vi "vibratome3 waveform gen.vi"(8 "error in":errorcluster, 9 "frequency(HZ)":dbl format="%#_13g", 10 "slice time":dbl format="%#_13g", 11 "ramp time(s)":dbl format="%#_13g") -> (0 "error out":errorcluster, 2 "vib wave":dbl[](graph))   [LabVIEW 2018]
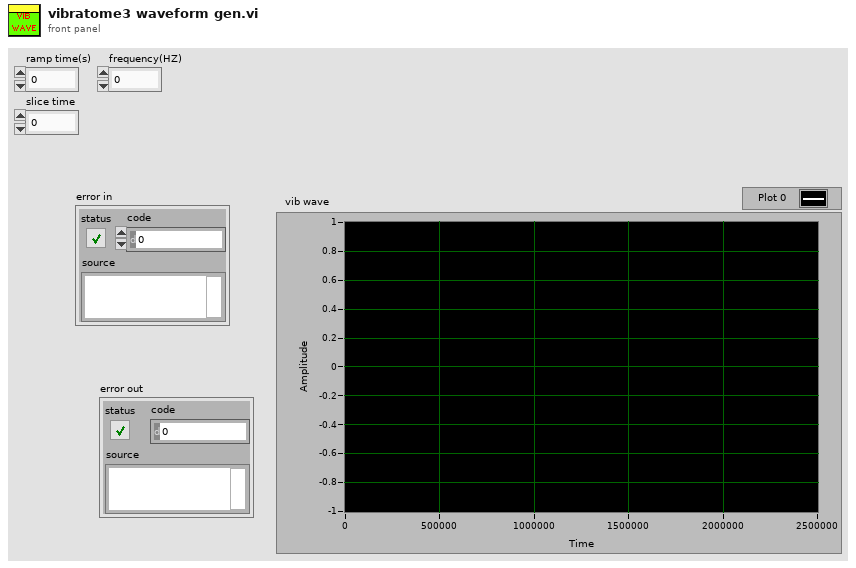
[diagram p1: front panel]
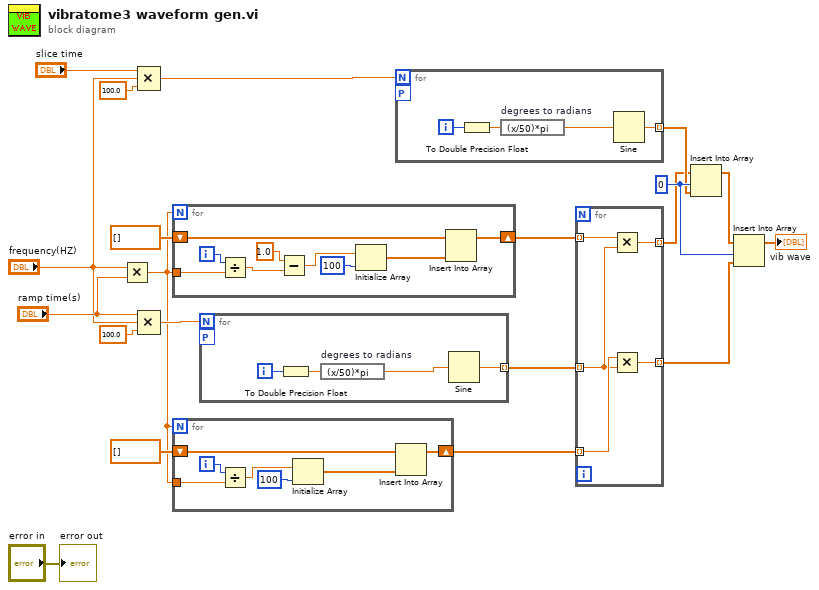
[diagram p0: block diagram]
diagram:
  w6 = 0 ("index")
  n1 = Multiply(x="frequency(HZ)", y="ramp time(s)") -> (x*y=w8:dbl)
  n2 = Compound Arithmetic op=MULTIPLY("slice time", "frequency(HZ)", 100.0) -> (w14:dbl)
  n3 = Compound Arithmetic op=MULTIPLY("ramp time(s)", "frequency(HZ)", 100.0) -> (w19:dbl)
  n4 = for {
    N: w8 -> [_]
    tunnel: w8 -> [w28]
    shift-right: [w24] -> w10
    shift-left: dbl[] [] -> [w25]
    i -> [w29]
    n5 = Divide(x=w29, y=w28) -> (x/y=w21:dbl)
    n6 = Subtract(x=1.0, y=w21) -> (x-y=w23:dbl)
    n7 = Initialize Array(w23, 100 ("dimension size")) -> (w26:dbl[])
    n8 = Insert Into Array(array=w25, new element=w26) -> (w24:dbl[])  [unwired: 1 in]
  }
  n9 = for {
    N: w8 -> [_]
    tunnel: w8 -> [w35]
    shift-right: [w30] -> w11
    shift-left: dbl[] [] -> [w31]
    i -> [w36]
    n10 = Divide(x=w36, y=w35) -> (x/y=w34:dbl)
    n11 = Initialize Array(w34, 100 ("dimension size")) -> (w32:dbl[])
    n12 = Insert Into Array(array=w31, new element=w32) -> (w30:dbl[])  [unwired: 1 in]
  }
  n13 = for {
    N: w19 -> [_]
    tunnel: [w37] -> w9 mode=indexing
    workers-P: _ -> [_]
    i -> [w40]
    n14 = To Double Precision Float(number=w40) -> (double precision float=w39:dbl)
    n15 = expression code="(x/50)*pi" "degrees to radians"(w39) -> (w38:dbl)
    n16 = Sine(x=w38) -> (sin(x)=w37:dbl)
  }
  n17 = for {
    N: w14 -> [_]
    tunnel: [w41] -> w5 mode=indexing
    workers-P: _ -> [_]
    i -> [w44]
    n18 = To Double Precision Float(number=w44) -> (double precision float=w43:dbl)
    n19 = expression code="(x/50)*pi" "degrees to radians"(w43) -> (w42:dbl)
    n20 = Sine(x=w42) -> (sin(x)=w41:dbl)
  }
  n21 = for {
    tunnel: w11 -> [w49] mode=indexing
    tunnel: w10 -> [w48] mode=indexing
    tunnel: w9 -> [w47] mode=indexing
    tunnel: [w46] -> w2 mode=indexing
    tunnel: [w45] -> w3 mode=indexing
    n22 = Multiply(x=w48, y=w47) -> (x*y=w45:dbl)
    n23 = Multiply(x=w49, y=w47) -> (x*y=w46:dbl)
  }
  n24 = Insert Into Array(array=w3, index=w6, new element=w5) -> (w7:dbl[])
  n25 = Insert Into Array(array=w7, index=w6, new element=w2) -> (→"vib wave":dbl[])
  "error out" <- "error in"
